vi "Stop Core.vi"(10 "final error code":i32, 11 "Controller in":refnum<class "Controller.lvclass">) -> (3 "Controller out":refnum<class "Controller.lvclass">)   [LabVIEW 2020, in "Controller.lvlib" / "Controller.lvclass"]
doc: "(<B>Filename</B>: Actor Framework.lvlib:Actor.lvclass:Stop Core.vi)\n\nDefines what the actor does before it stops. Use the <B>final error code</B> input to determine whether the actor shut down in response to an error.\n\nBy default, this method passes the Stop message along to all auto-stop nested actors. A descendant class may override this method to define additional behavior, such as shutting down any processes the actor initiated in its override of the Actor Core method."
uses:
  Controller.lvclass
  Controller.lvclass/Controller.ctl
  <vilib>/ActorFramework/Stop Msg/Stop Msg.lvclass/Stop Msg.ctl
  <vilib>/ActorFramework/Message Enqueuer/Message Enqueuer.lvclass/Message Enqueuer.ctl
  <vilib>/ActorFramework/Stop Msg/Send Emergency Stop.vi
  <vilib>/ActorFramework/Stop Msg/Send Normal Stop.vi
  <vilib>/ActorFramework/Message Enqueuer/Enqueue.vi
  <vilib>/ActorFramework/Message Enqueuer/Enqueue Critical.vi
  <vilib>/ActorFramework/Stop Msg/Stop Msg.lvclass
  C:/Program Files/National Instruments/LabVIEW 2020/vi.lib/ActorFramework/Message/Message.lvclass
  Main_UI/Main_UI Messages/Do UI Exit Msg/Do UI Exit Msg.lvclass
  <vilib>/ActorFramework/Message Priority Queue/Priority Enqueue.vi
  <vilib>/ActorFramework/Actor/Actor.lvclass
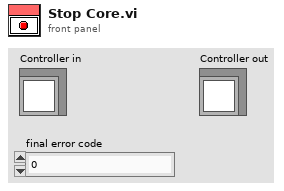
[diagram p1: front panel]
types:
  T1 = cluster{"Main UI Enqueuer":refnum<class "Message Enqueuer.lvclass">, "Log Enqueuer":refnum<class "Message Enqueuer.lvclass">, "NI6008 Enqueuer":refnum<class "Message Enqueuer.lvclass">, "AFG Enqueuer":refnum<class "Message Enqueuer.lvclass">, "Pulser Enqueuer":refnum<class "Message Enqueuer.lvclass">, "Scope Enqueuer":refnum<class "Message Enqueuer.lvclass">}
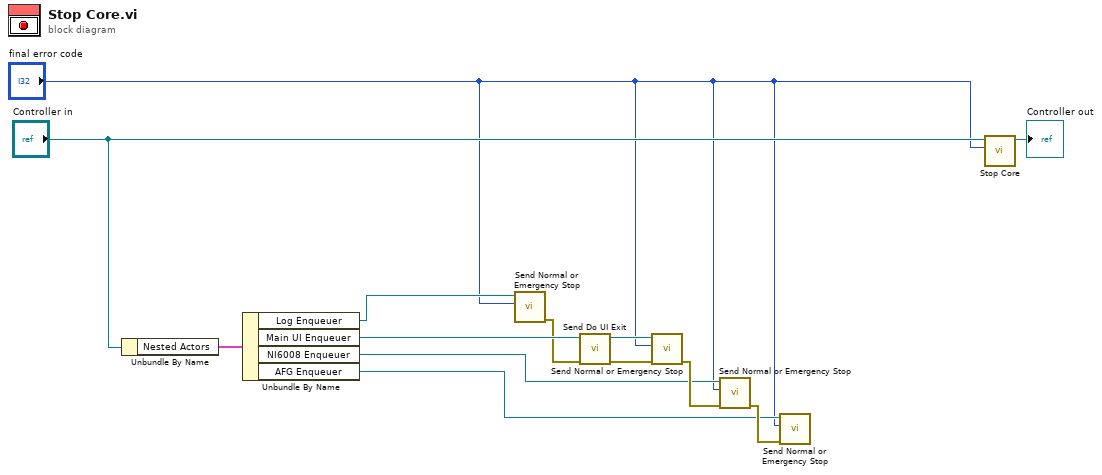
[diagram p0: block diagram]
diagram:
  n1 = Unbundle By Name("Controller in") -> ("Nested Actors"=w11:T1)
  n2 = Unbundle By Name(w11) -> ("Log Enqueuer"=w8:refnum<class "Message Enqueuer.lvclass">, "Main UI Enqueuer"=w10:refnum<class "Message Enqueuer.lvclass">, "NI6008 Enqueuer"=w4:refnum<class "Message Enqueuer.lvclass">, "AFG Enqueuer"=w2:refnum<class "Message Enqueuer.lvclass">)
  n3 = call <vilib>:"Send Normal or Emergency Stop.vi"("final error code"="final error code", "Message Enqueuer"=w8) -> ("error out"=w7:errorcluster)  [unwired: 9 in]
  n4 = call "Send Do UI Exit.vi"("error in (no error)"=w7, "Message Enqueuer"=w10) -> ("error out"=w6:errorcluster, "Message Enqueuer out"=w9:refnum<class "Message Enqueuer.lvclass">)  [unwired: 8 in]
  n5 = call <vilib>:"Send Normal or Emergency Stop.vi"("error in (no error)"=w6, "final error code"="final error code", "Message Enqueuer"=w9) -> ("error out"=w5:errorcluster)  [unwired: 8 in]
  n6 = call <vilib>:"Send Normal or Emergency Stop.vi"("error in (no error)"=w5, "final error code"="final error code", "Message Enqueuer"=w4) -> ("error out"=w3:errorcluster)  [unwired: 8 in]
  n7 = call <vilib>:"Send Normal or Emergency Stop.vi"("error in (no error)"=w3, "final error code"="final error code", "Message Enqueuer"=w2) -> ()  [unwired: 8 in, 1 out]
  n8 = call-parent "Stop Core.vi"("final error code"="final error code", "Actor in"="Controller in") -> ("Actor out"=→"Controller out":refnum<class "Controller.lvclass">)  [unwired: 9 in]
